vi "Obtain Session.vi"(0 "Session  Name ()":string, 5 "Limits File Path":path, 7 "Sequence File":refnum<k7>, 9 "Use Existing Test Numbers?":bool, 11 "error in (no error)":errorcluster) -> (4 "Session Handle":T1, 15 "error out":errorcluster)   [LabVIEW 2018, in "Test Number and Bin Generator.lvlib" / "Test Number and Bin Generator.lvclass"]
doc: "This function initializes the measurement\n\nPass the function a name to obtain an active measurement handle"
uses:
  Test Number and Bin Generator.lvclass
  Typedefs/Session Handle.ctl
  C:/Sequence Automation/Plugins/Sequence Automation Session.lvlibp/Sequence Automation Session.lvclass
  Test Number and Bin Generator.lvclass/Test Number and Bin Generator.ctl
  Plugins/Sequence Automation Session.lvlibp/Sequence Automation Session.lvclass
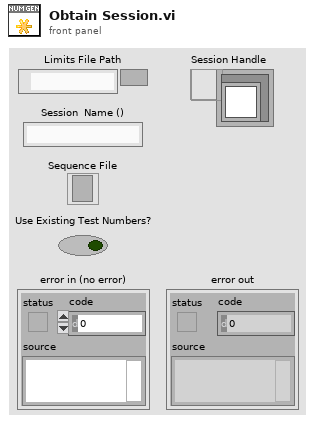
[diagram p1: front panel]
types:
  T1 = typedef "Test Number and Bin Generator.lvlib/Test Number and Bin Generator.lvclass/Session Handle.ctl" = refnum<data-value>
  T2 = typedef "Sequence Automation Session.lvlibp/Sequence Automation Session.lvclass/Session Handle.ctl" = refnum<data-value>
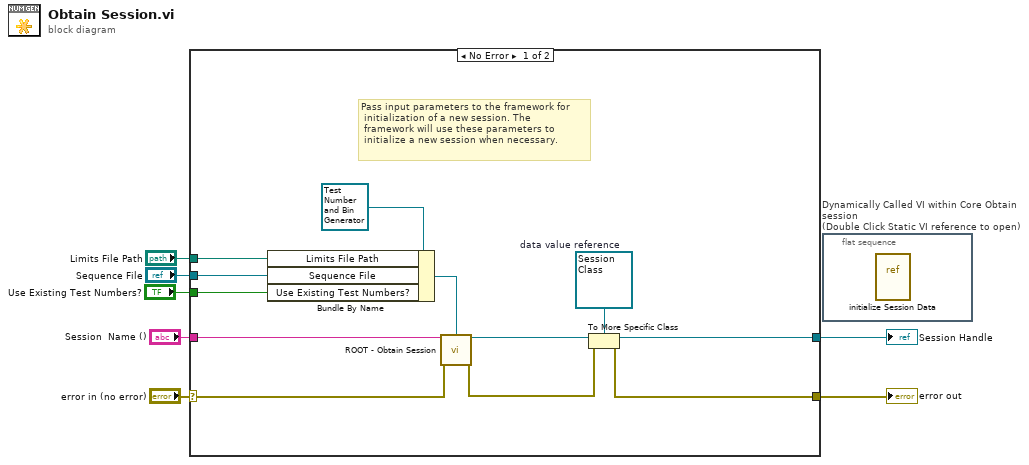
[diagram p0: block diagram]
diagram:
  n1 = case shown="No Error" "error in (no error)" {
    selector: "error in (no error)" -> [w18 w20]
    tunnel: [w15 w20] -> w6
    tunnel: [w17 _] -> w4
    tunnel: "Session  Name ()" -> [w19 _]
    tunnel: "Limits File Path" -> [w12 _]
    tunnel: "Sequence File" -> [w11 _]
    tunnel: "Use Existing Test Numbers?" -> [w10 _]
    frame No Error {
      w13 = refnum<data-value> refnum  # data value reference
      # "Pass input parameters to the framework for\n initialization of a new session. The\n framework will use these parameters to\n initialize a new session when necessary."
      n2 = Bundle By Name(cluster=refnum<class "Test Number and Bin Generator.lvclass"> refnum ("Test Number and Bin Generator.lvlib:Test Number and Bin Generator"), "Limits File Path"=w12, "Sequence File"=w11, "Use Existing Test Numbers?"=w10) -> (w9:refnum<class "Test Number and Bin Generator.lvclass">)
      n3 = call "ROOT - Obtain Session.vi"("Session Name ()"=w19, "OBJ - Session"=w9, "error in (no error)"=w18) -> ("Session Handle"=w14:T2, "error out"=w16:errorcluster)  [unwired: 10 in, 1 out]
      n4 = To More Specific Class(target class=w13, reference=w14, error in=w16) -> (specific class reference=w17:refnum<data-value>, error out=w15:errorcluster)
    }
    frame Error {
    }
  }
  "error out" <- w6
  "Session Handle" <- w4
  n5 = flat-sequence "Dynamically Called VI within Core Obtain session\n(Double Click Static VI reference to open)" {
    frame #0 {
      n6 = vi-ref "initialize Session Data.vi"() -> ()  [unwired: 1 out]
    }
  }
